vi "search for hook.vi"(10 "RobotDriveDevRef in":T1, 11 "Hook Found":bool) -> (0 "error out":errorcluster, 1 "Pixels to turn":dbl, 2 "RobotDriveDevRef out":T1, 3 "Move forward? S 5":bool, 4 "Hook found":bool, 5 "Hook Found In False Case 2":bool, 6 "Degrees to turn":dbl, 7 "Hook Center":dbl)   [LabVIEW 2016]
uses:
  <vilib>/Rock Robotics/WPI/RobotDrive/WPI_RobotDriveDevRef.ctl
  <vilib>/Rock Robotics/WPI/MotorControl/WPI_MotorControlDeviceRef.ctl
  <vilib>/Rock Robotics/WPI/MotorControl/WPI_MotorControlType.ctl
  <vilib>/Rock Robotics/SystemInterfaces/DIO/FPGA_DIOPWMChannel.ctl
  <vilib>/Rock Robotics/WPI/PWM/WPI_PWMDeadband.ctl
  <vilib>/Rock Robotics/Network Tables/NT Write Number.vi
  Robot Global Data.vi
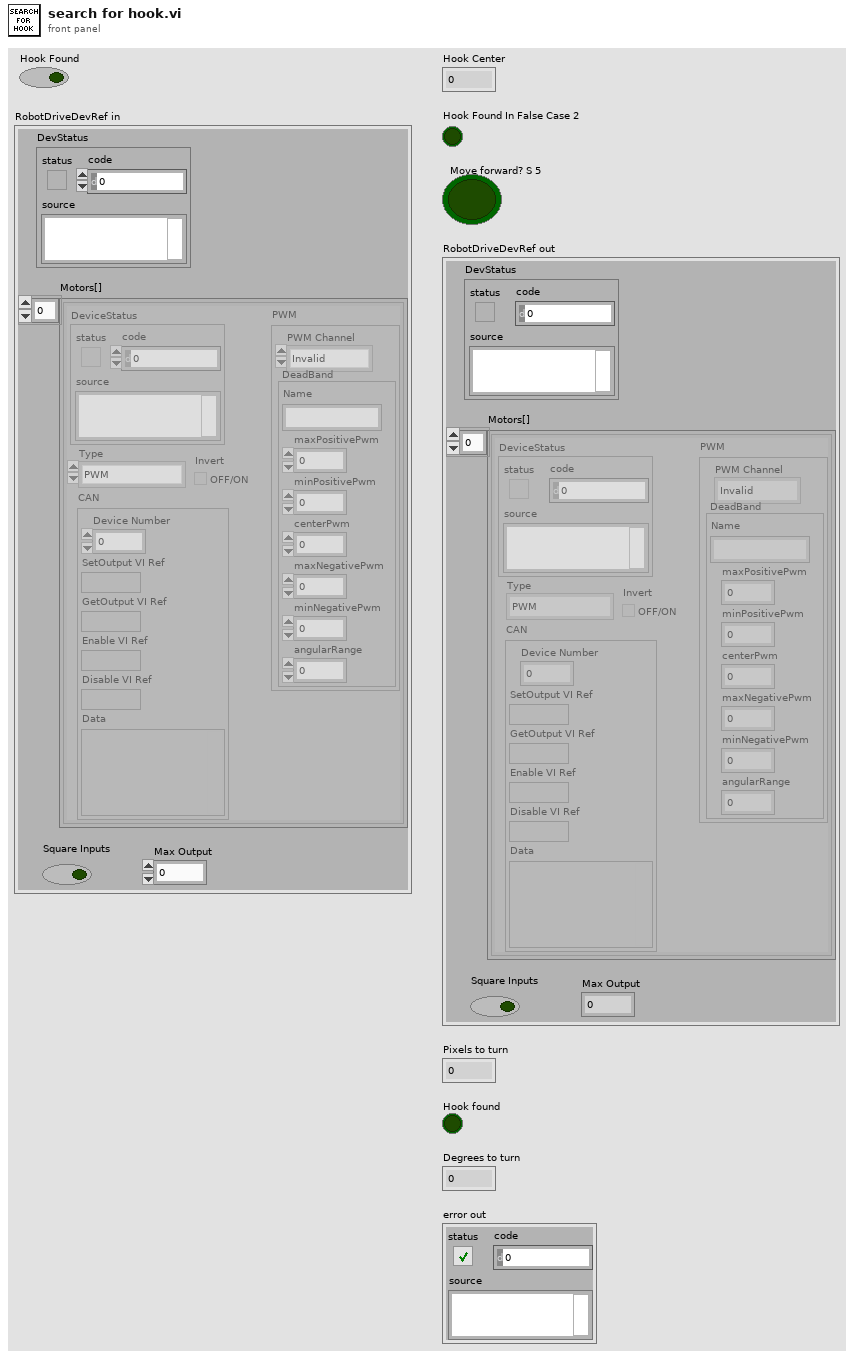
[diagram p1: front panel]
types:
  T1 = typedef "WPI_RobotDriveDevRef.ctl" = cluster{"DevStatus":errorcluster, "Motors[]":T2[], "Square Inputs":bool, "Max Output":dbl}
  T2 = typedef "WPI_MotorControlDeviceRef.ctl" = cluster{"DeviceStatus":errorcluster, "Type":T3, "PWM":cluster{"PWM Channel":T4, "DeadBand":T5}, "CAN":cluster{"Device Number":u8, "SetOutput VI Ref":variant, "GetOutput VI Ref":variant, "Enable VI Ref":variant, "Disable VI Ref":variant, "Data":variant}, "Invert":bool}
  T3 = typedef "WPI_MotorControlType.ctl" = enum16{"PWM", "CAN"}
  T4 = typedef "FPGA_DIOPWMChannel.ctl" = enum8{"PWM 0", "PWM 1", "PWM 2", "PWM 3", "PWM 4", "PWM 5", "PWM 6", "PWM 7", "PWM 8", "PWM 9", "PWM MXP 0", "PWM MXP 1", "PWM MXP 2", "PWM MXP 3", "PWM MXP 4", "PWM MXP 5", "PWM MXP 6", "PWM MXP 7", "PWM MXP 8", "PWM MXP 9", "Invalid"}
  T5 = typedef "WPI_PWMDeadband.ctl" = cluster{"Name":string, "maxPositivePwm":i32, "minPositivePwm":i32, "centerPwm":i32, "maxNegativePwm":i32, "minNegativePwm":i32, "angularRange":u16}
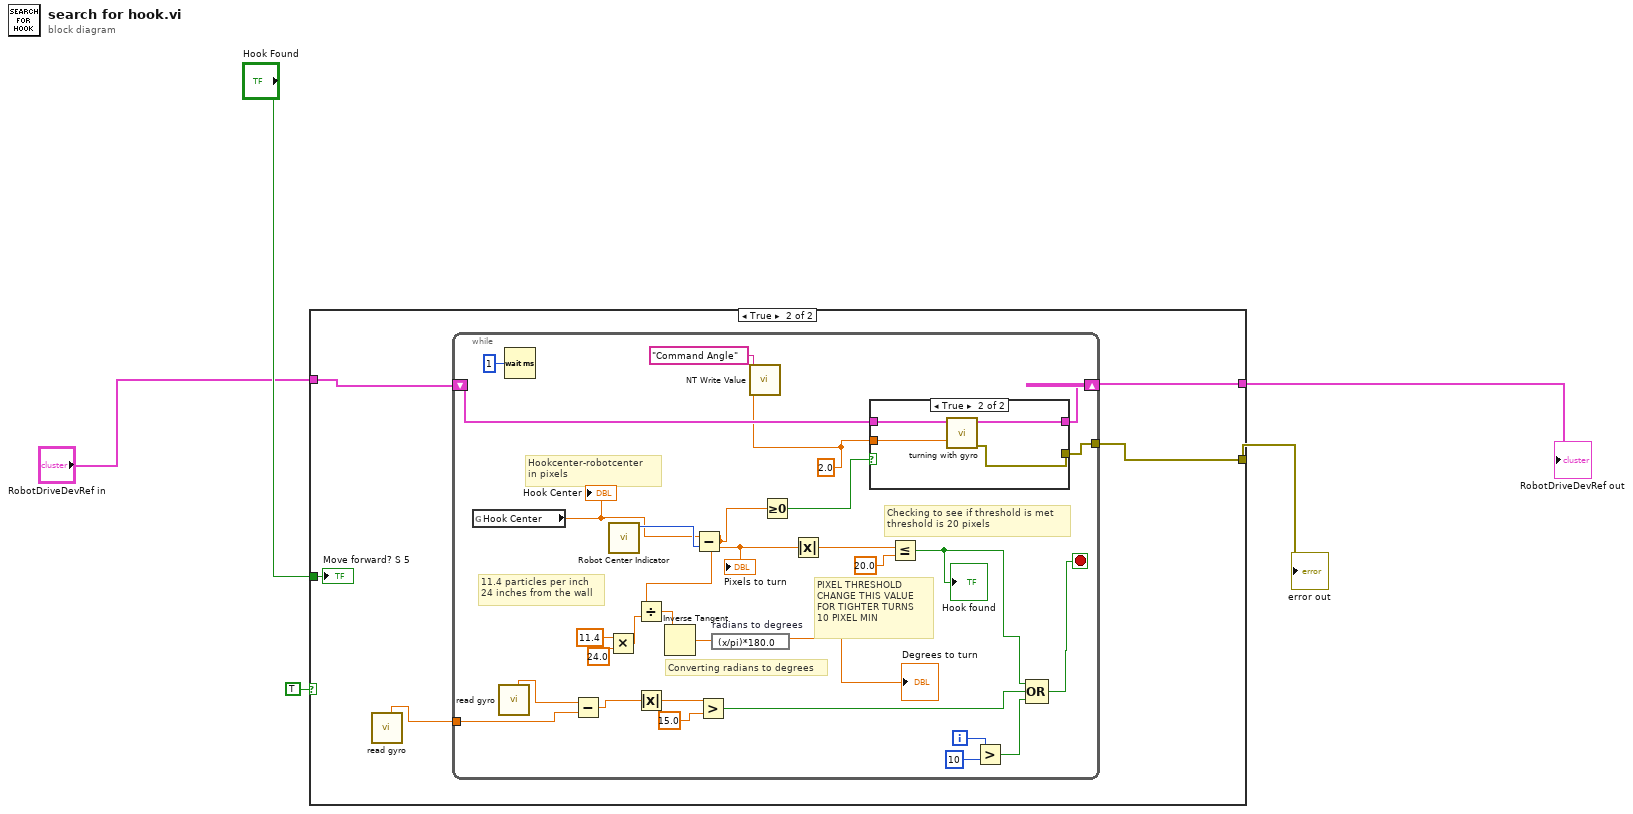
[diagram p0: block diagram]
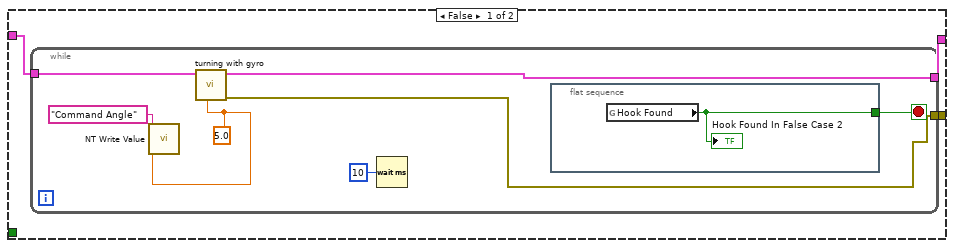
[diagram p2: hidden frame]
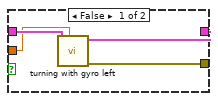
[diagram p3: hidden frame]
diagram:
  n1 = case shown="True" TRUE {
    tunnel: [w8 w21] -> w4
    tunnel: "RobotDriveDevRef in" -> [w7 w20]
    tunnel: [w6 w19] -> w3
    tunnel: "Hook Found" -> [_ w18]
    frame False {
      n2 = while {
        tunnel: [w14] -> w8
        tunnel: w7 -> [w13]
        tunnel: [w12] -> w6
        stop <- w15 stop-if-true
        w10 = 5.0 ("desired angle")
        n3 = call-poly <vilib>:"NT Write Value.vi"("Numeric"=w10, "Name"="Command Angle") -> ()  [unwired: 9 in, 1 out]
        n4 = call "turning with gyro.vi"("desired angle"=w10, "RobotDriveDevRef"=w13) -> ("error out"=w12:errorcluster, "RobotDriveDevRef 2"=w14:T1)  [unwired: 8 in]
        n5 = Wait (ms)(milliseconds to wait=u32 10) -> ()  [unwired: 1 out]
        n6 = flat-sequence {
          tunnel: [w16] -> w15
          frame #0 {
            n7 = global read "Robot Global Data.vi" "Hook Found"() -> (w16:bool)
            "Hook Found In False Case 2" <- w16
          }
        }
      }
    }
    frame True {
      n8 = call "read gyro.vi"() -> ("Angle 2"=w17:dbl)  [unwired: 10 in, 1 out]
      n9 = while {
        shift-right: [w46] -> w21
        shift-left: w20 -> [w47]
        tunnel: [w37] -> w19
        tunnel: w17 -> [w32]
        i -> [w24]
        stop <- w27 stop-if-true
        w28 = 2.0 ("Numeric")
        # "PIXEL THRESHOLD\nCHANGE THIS VALUE\nFOR TIGHTER TURNS \n10 PIXEL MIN"
        # "Checking to see if threshold is met\nthreshold is 20 pixels"
        # "Hookcenter-robotcenter \nin pixels"
        # "11.4 particles per inch\n24 inches from the wall"
        # "Converting radians to degrees"
        n10 = global read "Robot Global Data.vi" "Hook Center"() -> (w49:dbl)
        "Hook Center" <- w49
        n11 = call "read gyro.vi"() -> ("Angle 2"=w33:dbl)  [unwired: 10 in, 1 out]
        n12 = Wait (ms)(milliseconds to wait=u32 1) -> ()  [unwired: 1 out]
        n13 = Subtract(x=w33, y=w32) -> (x-y=w30:dbl)
        n14 = Multiply(x=11.4, y=24.0) -> (x*y=w41:dbl)
        n15 = call "Robot Center Indicator.vi"() -> ("Robot Center"=w50:i32)  [unwired: 10 in, 1 out]
        n16 = Absolute Value(x=w30) -> (abs(x)=w29:dbl)
        n17 = Subtract(x=w49, y=w50) -> (x-y=w38:dbl)
        "Pixels to turn" <- w38
        n18 = Divide(x=w38, y=w41) -> (x/y=w42:dbl)
        n19 = Inverse Tangent(1:w42) -> (0:w43:dbl)
        n20 = Greater?(x=w29, y=15.0) -> (0:w25:bool)
        n21 = expression code="(x/pi)*180.0" "radians to degrees"(w43) -> (→"Degrees to turn":dbl)
        n22 = call-poly <vilib>:"NT Write Value.vi"("Numeric"=w28, "Name"="Command Angle") -> ()  [unwired: 9 in, 1 out]
        n23 = Greater Or Equal To 0?(x=w38) -> (x >= 0?=w48:bool)
        n24 = Absolute Value(x=w38) -> (abs(x)=w45:dbl)
        n25 = case shown="True" w48 {
          tunnel: w47 -> [w54 w58]
          tunnel: [w53 w57] -> w46
          tunnel: w28 -> [w52 w56]
          tunnel: [w51 w55] -> w37
          frame False {
            n26 = call "turning with gyro left.vi"("desired angle"=w52, "RobotDriveDevRef"=w54) -> ("error out"=w51:errorcluster, "RobotDriveDevRef 2"=w53:T1)  [unwired: 7 in, 1 out]
          }
          frame True {
            n27 = call "turning with gyro.vi"("desired angle"=w56, "RobotDriveDevRef"=w58) -> ("error out"=w55:errorcluster, "RobotDriveDevRef 2"=w57:T1)  [unwired: 8 in]
          }
        }
        n28 = Less Or Equal?(x=w45, y=20.0) -> (x <= y?=w26:bool)
        "Hook found" <- w26
        n29 = Greater?(x=w24, y=10) -> (0:w23:bool)
        n30 = Compound Arithmetic op=OR(w26, w25, w23) -> (w27:bool)
      }
      "Move forward? S 5" <- w18
    }
  }
  "RobotDriveDevRef out" <- w4
  "error out" <- w3
